vi "Format Numeric String.vi"(10 "digits":u8=10, 11 "default value string":string) -> (3 "formatted default value string":string)   [LabVIEW 2014]
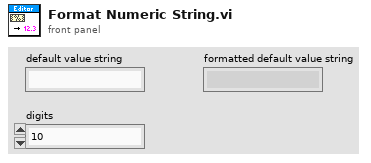
[diagram p1: front panel]
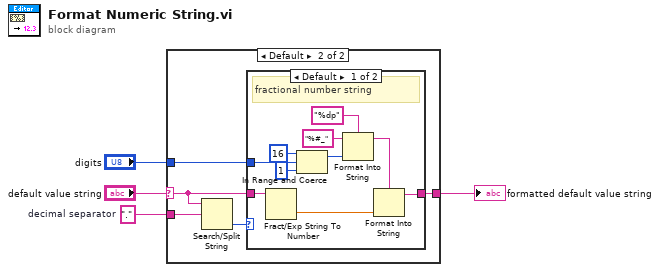
[diagram p0: block diagram]
diagram:
  w2 = "."  # decimal separator
  n1 = case shown="Default" "default value string" {
    selector: "default value string" -> [w5 w9]
    tunnel: [w5 w10] -> w4
    tunnel: w2 -> [_ w8]
    tunnel: "digits" -> [_ w6]
    frame "" {
    }
    frame Default {
      n2 = Search/Split String(string=w9, search string/char (-)=w8) -> (offset of match=w7:i32)  [unwired: 1 in, 2 out]
      n3 = case shown="Default" w7 {
        tunnel: w9 -> [w20 w21]
        tunnel: [w18 w21] -> w10
        tunnel: w6 -> [w11 _]
        frame Default {
          # "fractional number string"
          n4 = Fract/Exp String To Number(string=w20) -> (number=w19:dbl)  [unwired: 3 in, 1 out]
          n5 = In Range and Coerce(upper limit=u8 16, x=w11, lower limit=u8 1 ("y")) -> (coerced(x)=w12:u8)  [unwired: 1 out]
          n6 = Format Into String(format string="%dp", initial string="%#_", w12) -> (resulting string=w15:string)  [unwired: 1 in, 1 out]
          n7 = Format Into String(format string=w15, w19) -> (resulting string=w18:string)  [unwired: 2 in, 1 out]
        }
        frame -1 {
          # "integer --> no truncation"
        }
      }
    }
  }
  "formatted default value string" <- w4
